vi "util_find_system_path.vi"(8 "error in (no error)":errorcluster, 11 "relative_path_file":path) -> (0 "error out":errorcluster, 1 "found":bool, 2 "absolute_path":path, 3 "system_path":path)   [LabVIEW 2015, in "lv-bin.lvlib" / "v1.lvlib"]
uses:
  v1.lvlib
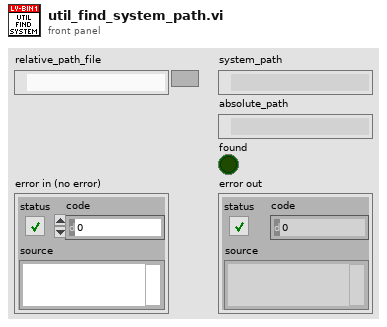
[diagram p1: front panel]
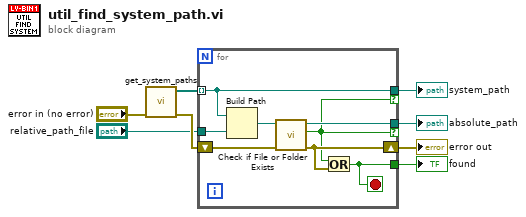
[diagram p0: block diagram]
diagram:
  n1 = call "get_system_paths.vi"("error in (no error)"="error in (no error)") -> ("error out"=w7:errorcluster, "paths []"=w6:path[])  [unwired: 9 in]
  n2 = for {
    tunnel: w6 -> [w12] mode=indexing
    shift-right: [w13] -> w4
    shift-left: w7 -> [w16]
    tunnel: "relative_path_file" -> [w14]
    tunnel: [w12] -> w3 if=w10
    tunnel: [w11] -> w2 if=w10
    tunnel: [w9] -> w1
    stop <- w9 stop-if-true
    n3 = Build Path(base path=w12, name or relative path=w14) -> (appended path=w15:path)
    n4 = call <vilib>:"Check if File or Folder Exists.vi"("error in (no error)"=w16, "path"=w15) -> ("error out"=w13:errorcluster, "file or folder exists?"=w10:bool, "dup path"=w11:path)  [unwired: 7 in]
    n5 = Or(x=w10, y=w13) -> (x .or. y?=w9:bool)
  }
  "error out" <- w4
  "absolute_path" <- w2
  "system_path" <- w3
  "found" <- w1
